vi "RandU32.vi"(3 "Limit b":u32=1 caption="Limit b (1)", 5 "Limit a":u32 caption="Limit a (0)") -> (1 "Random number":u32)   [LabVIEW 2017, in "GPNumeric.lvlib"]
doc: "Produces a <B>Random number</B> between <B>Limit a</B> and <B>Limit b</B>.\n\nIt doesn't matter which of <B>Limit a</B> and <B>Limit b</B> is highest, only the range is considered. Both limits are included in the range of random numbers.\n\nThis VI is polymorphic, right click on it to select the data type.\n\nThis VI is inlined.\n\nSteen Schmidt\nGPower\n5/4 2014"
uses:
  GPNumeric.lvlib
panel:
  # "Copyright © 2014\nGPower\nSee enclosed license file for terms and conditions"
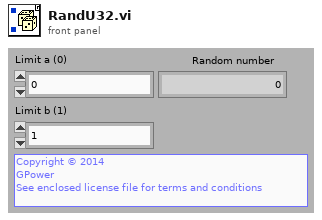
[diagram p1: front panel]
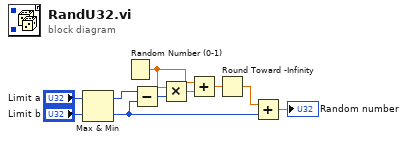
[diagram p0: block diagram]
diagram:
  n1 = Max & Min(x="Limit a", y="Limit b") -> (max(x,y)=w6:u32, min(x,y)=w5:u32)
  n2 = Random Number (0-1)() -> (number: 0 to 1=w2:dbl)
  n3 = Subtract(x=w6, y=w5) -> (x-y=w1:u32)
  n4 = Multiply(x=w2, y=w1) -> (x*y=w4:dbl)
  n5 = Add(x=w2, y=w4) -> (x+y=w3:dbl)
  n6 = Round Toward -Infinity(1:w3) -> (0:w7:dbl)
  n7 = Add(x=w7, y=w5) -> (x+y=→"Random number":dbl)
